vi "Change View.vi"(5 "Boolean in":refnum<vi>, 7 "VI Refnum":refnum<vi>, 8 "error in (no error)":errorcluster, 10 "Required View":string) -> (0 "error out":errorcluster)   [LabVIEW 2018]
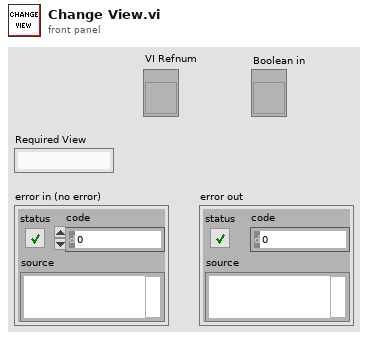
[diagram p1: front panel]
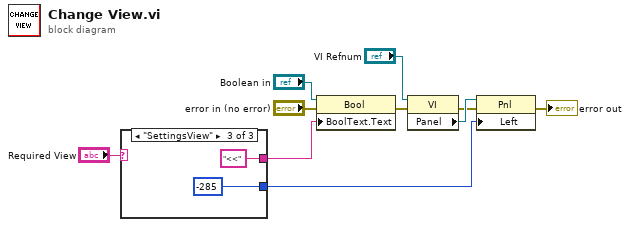
[diagram p0: block diagram]
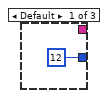
[diagram p2: hidden frame]
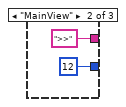
[diagram p3: hidden frame]
diagram:
  n1 = case shown="\"SettingsView\"" "Required View" {
    tunnel: [12 ("Position:Left") 12 ("Position:Left") -285 ("Position:Left")] -> w4
    tunnel: [_ ">>" ("Boolean Text.Text") "<<" ("Boolean Text.Text")] -> w7
    frame Default {
    }
    frame "MainView" {
    }
    frame "SettingsView" {
    }
  }
  n2 = property on="Property Node" class="Bool"(reference="Boolean in", error in="error in (no error)", "BoolText.Text"=w7) -> (error out=w3:errorcluster)  [unwired: 1 out]
  n3 = property on="Property Node" class="VI"(reference="VI Refnum", error in=w3) -> (error out=w2:errorcluster, "Panel"=w5:refnum<vi>)  [unwired: 1 out]
  n4 = property class="Pnl"(reference=w5, error in=w2, "Left"=w4) -> (error out=→"error out":errorcluster)  [unwired: 1 out]
